vi "ObjectDecorator_Init.vi"(8 "error in (no error)":errorcluster, 10 "Object":refnum<class "Object.lvclass">, 11 "object in":refnum<class "ObjectDecorator.lvclass">) -> (0 "error out":errorcluster, 3 "object out":refnum<class "ObjectDecorator.lvclass">)   [LabVIEW 2020, in "ObjectDecorator.lvclass"]
uses:
  ObjectDecorator.lvclass
  ObjectDecorator.lvclass/ObjectDecorator.ctl
  Object_interface/Object.lvclass
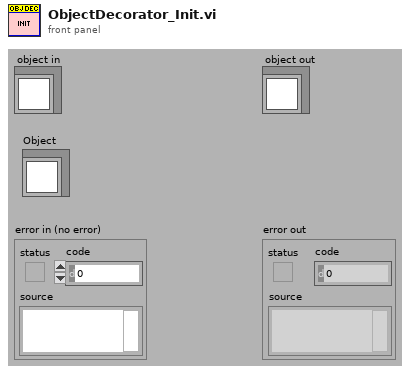
[diagram p1: front panel]
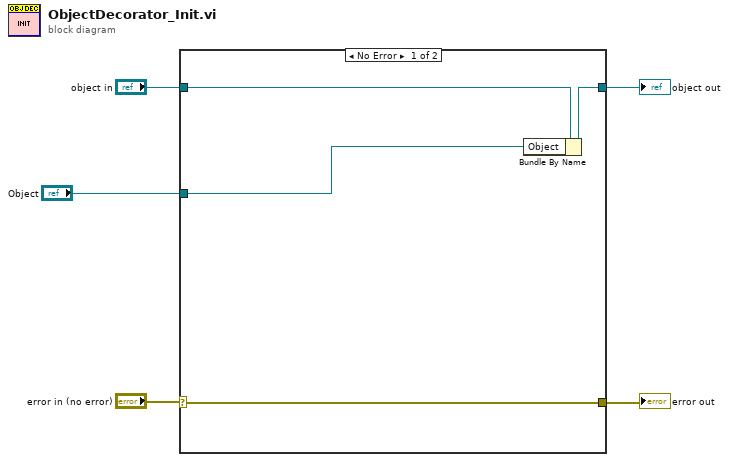
[diagram p0: block diagram]
diagram:
  n1 = case shown="No Error" "error in (no error)" {
    selector: "error in (no error)" -> [w7 w10]
    tunnel: "object in" -> [w9 w11]
    tunnel: [w8 w11] -> w4
    tunnel: [w7 w10] -> w2
    tunnel: "Object" -> [w6 _]
    frame No Error {
      n2 = Bundle By Name(cluster=w9, "Object"=w6) -> (w8:refnum<class "ObjectDecorator.lvclass">)
    }
    frame Error {
    }
  }
  "object out" <- w4
  "error out" <- w2
